vi "OVERIDE SOFT LIMITS.vi"(11 "Override Limit Switches?":bool) -> ()   [LabVIEW 2020]
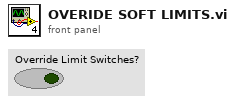
[diagram p1: front panel]
types:
  T1 = typedef "WPI_MotorControlDeviceRef.ctl" = cluster{"DeviceStatus":errorcluster, "Type":T2, "PWM":cluster{"PWM Channel":T3, "DeadBand":T4}, "CAN":cluster{"Device Number":u8, "SetOutput VI Ref":variant, "GetOutput VI Ref":variant, "Enable VI Ref":variant, "Disable VI Ref":variant, "Data":variant}, "Invert":bool, "DIO PWM":cluster{"PWM \"Enable\" Channel":T3, "DIOChannel":T5, "PWM Rate":dbl}}
  T2 = typedef "WPI_MotorControlType.ctl" = enum16{"PWM", "CAN", "DIO PWM"}
  T3 = typedef "FPGA_DIOPWMChannel.ctl" = enum8{"PWM 0", "PWM 1", "PWM 2", "PWM 3", "PWM 4", "PWM 5", "PWM 6", "PWM 7", "PWM 8", "PWM 9", "PWM MXP 0", "PWM MXP 1", "PWM MXP 2", "PWM MXP 3", "PWM MXP 4", "PWM MXP 5", "PWM MXP 6", "PWM MXP 7", "PWM MXP 8", "PWM MXP 9", "Invalid"}
  T4 = typedef "WPI_PWMDeadband.ctl" = cluster{"Name":string, "maxPositivePwm":i32, "minPositivePwm":i32, "centerPwm":i32, "maxNegativePwm":i32, "minNegativePwm":i32, "angularRange":u16}
  T5 = typedef "FPGA_DIOChannel.ctl" = enum8{"DIO 0", "DIO 1", "DIO 2", "DIO 3", "DIO 4", "DIO 5", "DIO 6", "DIO 7", "DIO 8", "DIO 9", "DIO MXP 0", "DIO MXP 1", "DIO MXP 2", "DIO MXP 3", "DIO MXP 4", "DIO MXP 5", "DIO MXP 6", "DIO MXP 7", "DIO MXP 8", "DIO MXP 9", "DIO MXP 10", "DIO MXP 11", "DIO MXP 12", "DIO MXP 13", "DIO MXP 14", "DIO MXP 15", "SPI Port CS1", "SPI Port CS2", "SPI Port CS3", "SPI Port MISO", "SPI Port MOSI", "Invalid"}
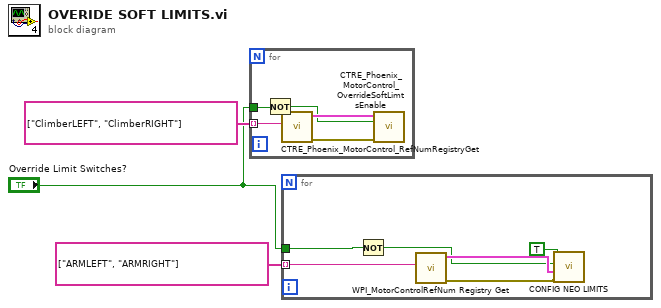
[diagram p0: block diagram]
diagram:
  n1 = for {
    tunnel: string[] ["ClimberLEFT", "ClimberRIGHT"] ("Phoenix motor refname") -> [w8] mode=indexing
    tunnel: "Override Limit Switches?" -> [w7]
    n2 = Not(x=w7) -> (.not. x?=w4:bool)
    n3 = call <vilib>:"CTRE_Phoenix_MotorControl_RefNumRegistryGet.vi"("refnum name"=w8) -> ("error out"=w5:errorcluster, "PhoenixMotorControlDevRef"=w6:T1)  [unwired: 9 in]
    n4 = call <vilib>:"CTRE_Phoenix_MotorControl_OverrideSoftLimtsEnable.vi"("PhoenixMotorControlDevRef"=w6, "Override Soft Limit Enable?"=w4, "error in (no error)"=w5) -> ()  [unwired: 11 in, 2 out]
  }
  n5 = for {
    tunnel: string[] ["ARMLEFT", "ARMRIGHT"] ("Phoenix motor refname") -> [w14] mode=indexing
    tunnel: "Override Limit Switches?" -> [w10]
    n6 = Not(x=w10) -> (.not. x?=w9:bool)
    n7 = call <vilib>:"WPI_MotorControlRefNum Registry Get.vi"("refnum name"=w14) -> ("error out"=w12:errorcluster, "MotorControlDevRef"=w13:T1)  [unwired: 9 in]
    n8 = call "CONFIG NEO LIMITS.vi"("error in (no error)"=w12, "MotorControlDeviceRef in"=w13, "Enable SOFT LIMIT? (T)"=w9, "Enable HARD LIMIT? (T)"=TRUE) -> ()  [unwired: 6 in, 2 out]
  }
